vi "EvaluateNode.vi"(8 "error in (no error)":errorcluster, 10 "ToEvaluate in":refnum<data-value>, 11 "MultiTree in":refnum<class "MultiTree.lvclass">) -> (0 "error out":errorcluster, 2 "ToEvaluate out":refnum<data-value>, 3 "MultiTree out":refnum<class "MultiTree.lvclass">)   [LabVIEW 2014, in "MultiTree.lvlib" / "MultiTree.lvclass"]
uses:
  <userlib>/AdvancedDataStructures/ClassBased/MultiTree/MultiTree.lvclass
  <userlib>/AdvancedDataStructures/ClassBased/MultiTreeNode/MultiTreeNode.lvclass
  <userlib>/AdvancedDataStructures/ClassBased/MultiTreeNode/MultiTreeNode.lvclass/MultiTreeNode.ctl
  <vilib>/Analysis/baseanly.llb/Mean (DBL).vi
  <userlib>/AdvancedDataStructures/ClassBased/Common/BasicSortedList/BasicSortedNode/BasicSortedNode.lvclass
  <vilib>/Analysis/NI_AALBase.lvlib
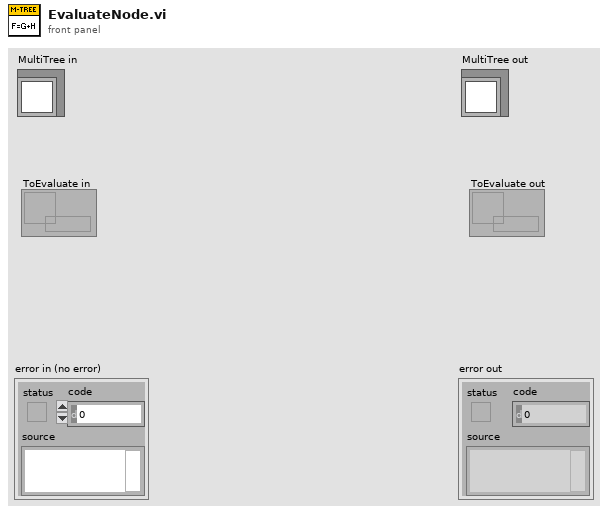
[diagram p1: front panel]
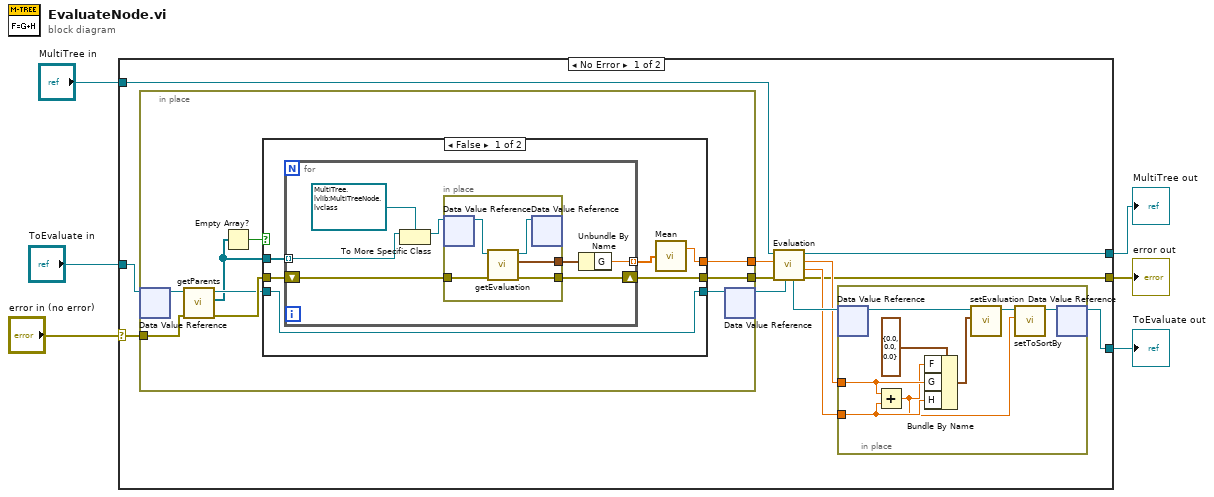
[diagram p0: block diagram]
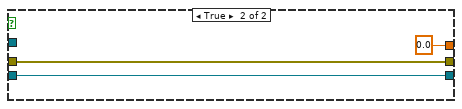
[diagram p2: hidden frame]
diagram:
  n1 = case shown="No Error" "error in (no error)" {
    selector: "error in (no error)" -> [w11 w59]
    tunnel: [w10 w59] -> w5
    tunnel: [w7 w58] -> w3
    tunnel: "MultiTree in" -> [w12 w58]
    tunnel: [w9 w57] -> w2
    tunnel: "ToEvaluate in" -> [w8 w57]
    frame No Error {
      n2 = in-place {
        in-place-border: w11 -> [w29]
        in-place-border: [w28] -> w18
        in-place-border: [w27] -> w17
        n3 = in-place-dvr #1(w8) -> (w31:refnum<class "MultiTreeNode.lvclass">)  [unwired: 1 out]
        n4 = call <userlib>:"getParents.vi"("error in (no error)"=w29, "MultiTreeNode in"=w31) -> ("error out"=w34:errorcluster, "Parents"=w32:refnum<data-value>[], "MultiTreeNode out"=w33:refnum<class "MultiTreeNode.lvclass">)  [unwired: 7 in]
        n5 = Empty Array?(array=w32) -> (empty?=w35:bool)
        n6 = case shown="False" w35 {
          tunnel: w34 -> [w39 w55]
          tunnel: w33 -> [w40 w56]
          tunnel: w32 -> [w41 _]
          tunnel: [w40 w56] -> w30
          tunnel: [w38 w55] -> w28
          tunnel: [w36 0.0 ("Parents G")] -> w27
          frame False {
            n7 = for {
              tunnel: w41 -> [w48] mode=indexing
              tunnel: [w42] -> w37 mode=indexing
              shift-right: [w44] -> w38
              shift-left: w39 -> [w45]
              n8 = To More Specific Class(target class=refnum<data-value> refnum ("data value reference"), reference=w48) -> (specific class reference=w46:refnum<data-value>)  [unwired: 1 in, 1 out]
              n9 = in-place {
                in-place-border: w45 -> [w52]
                in-place-border: [w51] -> w44
                in-place-border: [w50] -> w43
                n10 = in-place-dvr #2(w46) -> (w53:refnum<class "MultiTreeNode.lvclass">)  [unwired: 1 out]
                n11 = call <userlib>:"getEvaluation.vi"("error in (no error)"=w52, "MultiTreeNode in"=w53) -> ("error out"=w51:errorcluster, "evaluation"=w50:cluster{"F":dbl, "G":dbl, "H":dbl}, "MultiTreeNode out"=w49:refnum<class "MultiTreeNode.lvclass">)  [unwired: 7 in]
                n12 = in-place-dvr #2(w49) -> ()  [unwired: 2 out]
              }
              n13 = Unbundle By Name(w43) -> ("G"=w42:dbl)
            }
            n14 = call-poly <vilib>:"Mean.vi"("X"=w37) -> ("mean"=w36:dbl)  [unwired: 1 out]
          }
          frame True {
          }
        }
        n15 = in-place-dvr #1(w30) -> (w16:refnum<data-value>)  [unwired: 1 out]
      }
      n16 = call-dynamic "Evaluation.vi"("ToEvaluate in"=w16, "error in (no error)"=w18, "Parents G"=w17, "MultiTree in"=w12) -> ("error out"=w10:errorcluster, "H"=w13:dbl, "G"=w14:dbl, "MultiTree out"=w7:refnum<class "MultiTree.lvclass">, "ToEvaluate out"=w15:refnum<data-value>)  [unwired: 3 in]
      n17 = in-place {
        in-place-border: w14 -> [w24]
        in-place-border: w13 -> [w23]
        n18 = in-place-dvr #3(w15) -> (w26:refnum<class "MultiTreeNode.lvclass">)  [unwired: 1 out]
        n19 = Add(x=w24, y=w23) -> (x+y=w19:dbl)
        n20 = Bundle By Name(cluster=cluster{"F":dbl, "G":dbl, "H":dbl} {"F"=0.0, "G"=0.0, "H"=0.0} ("evaluation"), "F"=w19, "G"=w24, "H"=w23) -> (w22:cluster{"F":dbl, "G":dbl, "H":dbl})
        n21 = call <userlib>:"setEvaluation.vi"("evaluation"=w22, "MultiTreeNode in"=w26) -> ("MultiTreeNode out"=w21:refnum<class "MultiTreeNode.lvclass">)  [unwired: 8 in, 1 out]
        n22 = call <userlib>:"setToSortBy.vi"("ToSortBy"=w19, "BasicSortedNode in"=w21) -> ("BasicSortedNode out"=w20:refnum<class "MultiTreeNode.lvclass">)  [unwired: 8 in, 1 out]
        n23 = in-place-dvr #3(w20) -> (w9:refnum<data-value>)  [unwired: 1 out]
      }
    }
    frame Error {
    }
  }
  "error out" <- w5
  "MultiTree out" <- w3
  "ToEvaluate out" <- w2
